vi "Get Wheel Information_Steering.vi"(8 "error in (no error)":errorcluster, 11 "steering wheel in":refnum<class "NI_Robotics_Steering Wheel.lvclass">) -> (0 "error out":errorcluster, 1 "wheel name":string, 2 "wheel parameters":T3={"wheel radius"=1.0, "gear ratio"=1.0, "forward rotation direction"=0} {"forward rotation direction" items=["Clockwise", "Counterclockwise"]}, 3 "steering wheel out":refnum<class "NI_Robotics_Steering Wheel.lvclass">, 4 "motor communication":refnum<class "NI_Robotics_Motor Communication.lvclass">, 5 "steering parameters":T1={"steering gear ratio"=1.0, "motor angle offset (rad)"=0.0, "steering angle range"={"min steering angle (rad)"=-3.14159, "max steering angle (rad)"=3.141592653589793}}, 6 "steering motor communication":refnum<class "NI_Robotics_Motor Communication.lvclass">)   [LabVIEW 2017, in "NI_Robotics_Steering Wheel.lvclass"]
doc: "Returns information, such as <B>wheel radius</B> and <B>gear ratio</B>, for the wheel you specify. You must manually select the polymorphic instance to use."
uses:
  <vilib>/robotics/Steering/Steering Wheel/NI_Robotics_Steering Wheel.lvclass
  c:/Program Files (x86)/National Instruments/LabVIEW 2017/vi.lib/robotics/Steering/Wheel/NI_Robotics_Wheel.lvclass
  <vilib>/robotics/Steering/Wheel/Wheel Parameters.ctl
  <vilib>/robotics/Steering/Wheel/Rotation Direction.ctl
  <vilib>/robotics/Steering/Steering Wheel/Steering Wheel Parameters.ctl
  <vilib>/robotics/Steering/Steering Wheel/Steering Angle Range.ctl
  <vilib>/robotics/Actuation/Motor Communication/NI_Robotics_Motor Communication.lvclass
  <vilib>/robotics/Steering/Steering Wheel/NI_Robotics_Steering Wheel.lvclass/NI_Robotics_Steering Wheel.ctl
  <vilib>/robotics/Steering/Wheel/NI_Robotics_Wheel.lvclass/NI_Robotics_Wheel.ctl
  <vilib>/Analysis/coordinate.llb/Wrap Angle.vi
  <vilib>/Analysis/coordinate.llb/Wrap Angle (scalar).vi
  <vilib>/robotics/Steering/Wheel/NI_Robotics_Wheel.lvclass
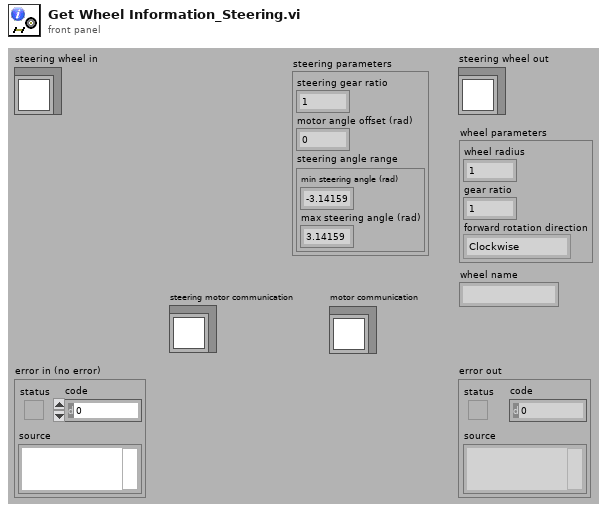
[diagram p1: front panel]
types:
  T1 = typedef "NI_Robotics_Steering Wheel.lvclass/Steering Wheel Parameters.ctl" = cluster{"steering gear ratio":dbl, "motor angle offset (rad)":dbl, "steering angle range":T2}
  T2 = typedef "NI_Robotics_Steering Wheel.lvclass/Steering Angle Range.ctl" = cluster{"min steering angle (rad)":dbl, "max steering angle (rad)":dbl}
  T3 = typedef "NI_Robotics_Wheel.lvclass/Wheel Parameters.ctl" = cluster{"wheel radius":dbl, "gear ratio":dbl, "forward rotation direction":T4}
  T4 = typedef "NI_Robotics_Wheel.lvclass/Rotation Direction.ctl" = u16
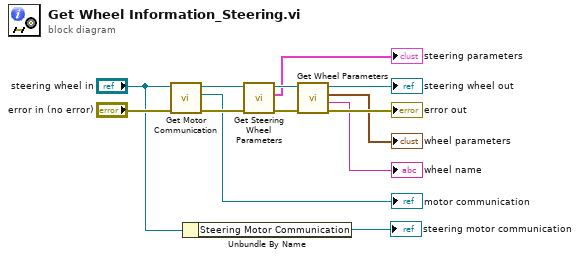
[diagram p0: block diagram]
diagram:
  n1 = call <vilib>:"Get Motor Communication.vi"("error in (no error)"="error in (no error)", "wheel in"="steering wheel in") -> ("error out"=w6:errorcluster, "motor communication"=→"motor communication":refnum<class "NI_Robotics_Motor Communication.lvclass">, "wheel out"=w8:refnum<class "NI_Robotics_Steering Wheel.lvclass">)  [unwired: 7 in]
  n2 = Unbundle By Name("steering wheel in") -> ("Steering Motor Communication"=→"steering motor communication":refnum<class "NI_Robotics_Motor Communication.lvclass">)
  n3 = call <vilib>:"Get Steering Wheel Parameters.vi"("error in (no error)"=w6, "steering wheel in"=w8) -> ("error out"=w5:errorcluster, "steering parameters"=→"steering parameters":T1, "steering wheel out"=w7:refnum<class "NI_Robotics_Steering Wheel.lvclass">)  [unwired: 7 in]
  n4 = call <vilib>:"Get Wheel Parameters.vi"("error in (no error)"=w5, "wheel in"=w7) -> ("error out"=→"error out":errorcluster, "wheel name"=→"wheel name":string, "wheel parameters"=→"wheel parameters":T3, "wheel out"=→"steering wheel out":refnum<class "NI_Robotics_Steering Wheel.lvclass">)  [unwired: 6 in]
